vi "Simulation Configuration Read.vi"(8 "error in (no error)":errorcluster, 10 "configuration":path=path "simulation configuration.ini", 11 "simulation configuration":T1={"maxTime"=5.0, "enableVisualization"=TRUE, "statechart"=path "iRobot Navigation State Machine.vi", "environment"=path "iRobot Navigation State Machine.vi", "record"=path "Simulation Record.xml", "autograde?"=TRUE, "interactive?"=FALSE, "feedback mode"=enum."debug navigation"}) -> (0 "error out":errorcluster, 3 "simulation configuration":T1={"maxTime"=5.0, "enableVisualization"=TRUE, "statechart"=path "iRobot Navigation State Machine.vi", "environment"=path "iRobot Navigation State Machine.vi", "record"=path "Simulation Record.xml", "autograde?"=TRUE, "interactive?"=FALSE, "feedback mode"=enum."debug navigation"})   [LabVIEW 2013]
uses:
  CyberSim interface/Simulation Configuration.ctl
  autograder/feedbackMode.ctl
  <vilib>/Utility/config.llb/Read Key (Path).vi
  <vilib>/Utility/config.llb/Read Key (U32).vi
  <vilib>/Utility/config.llb/NI_LVConfig.lvlib
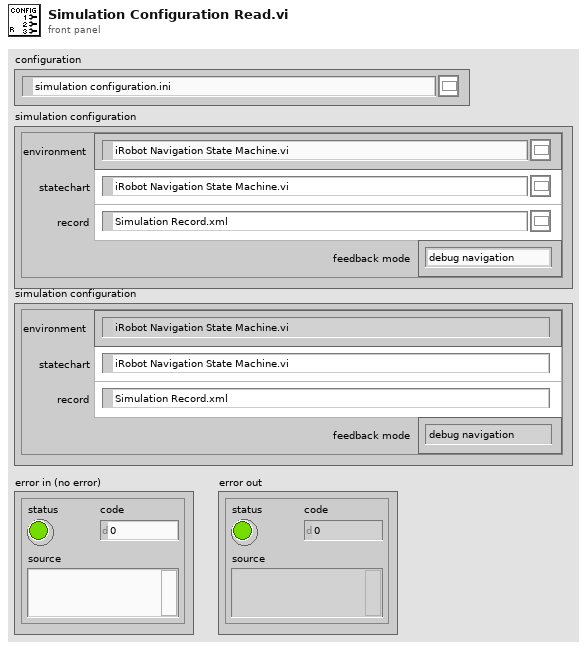
[diagram p1: front panel]
types:
  T1 = typedef "Simulation Configuration.ctl" = cluster{"maxTime":sgl, "enableVisualization":bool, "statechart":path, "environment":path, "record":path, "autograde?":bool, "interactive?":bool, "feedback mode":T2}
  T2 = typedef "feedbackMode.ctl" = enum32{"debug navigation", "debug hill climb", "autograde navigation", "autograde hill climb"}
  T3 = typedef "NI_LVConfig.lvlib/Config Data RefNum.ctl" = refnum<k1>
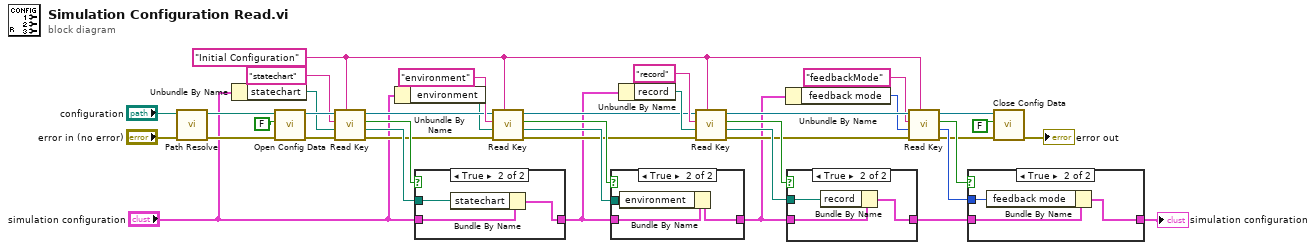
[diagram p0: block diagram]
diagram:
  w13 = "Initial Configuration" ("section")
  n1 = call "Path Resolve.vi"("Error In"="error in (no error)", "absolute or relative path"="configuration") -> ("Error Out"=w37:errorcluster, "resolved path"=w39:path)  [unwired: 8 in]
  n2 = Unbundle By Name("simulation configuration") -> ("statechart"=w21:path)
  n3 = call <vilib>:"Open Config Data.vi"("error in (no error)"=w37, "create file if necessary (T)"=FALSE, "configuration file path"=w39) -> ("error out"=w36:errorcluster, "refnum"=w35:T3)  [unwired: 6 in, 1 out]
  n4 = call-poly <vilib>:"Read Key.vi"("section"=w13, "error in (no error)"=w36, "default value"=w21, "key"="statechart" ("string key"), "refnum"=w35) -> ("error out"=w23:errorcluster, "value"=w31:path, "found?"=w32:bool, "refnum out"=w24:T3)  [unwired: 3 in]
  n5 = Unbundle By Name("simulation configuration") -> ("environment"=w20:path)
  n6 = case shown="True" w32 {
    tunnel: w31 -> [_ w43]
    tunnel: "simulation configuration" -> [w40 w42]
    tunnel: [w40 w41] -> w2
    frame False {
    }
    frame True {
      n7 = Bundle By Name(cluster=w42, "statechart"=w43) -> (w41:T1)
    }
  }
  n8 = call-poly <vilib>:"Read Key.vi"("section"=w13, "error in (no error)"=w23, "default value"=w20, "key"="environment" ("string key"), "refnum"=w24) -> ("error out"=w3:errorcluster, "value"=w29:path, "found?"=w30:bool, "refnum out"=w4:T3)  [unwired: 3 in]
  n9 = case shown="True" w30 {
    tunnel: w29 -> [_ w47]
    tunnel: w2 -> [w44 w46]
    tunnel: [w44 w45] -> w1
    frame False {
    }
    frame True {
      n10 = Bundle By Name(cluster=w46, "environment"=w47) -> (w45:T1)
    }
  }
  n11 = Unbundle By Name(w2) -> ("record"=w18:path)
  n12 = call-poly <vilib>:"Read Key.vi"("section"=w13, "error in (no error)"=w3, "default value"=w18, "key"="record", "refnum"=w4) -> ("error out"=w14:errorcluster, "value"=w16:path, "found?"=w17:bool, "refnum out"=w15:T3)  [unwired: 3 in]
  n13 = Unbundle By Name(w1) -> ("feedback mode"=w11:T2)
  n14 = case shown="True" w17 {
    tunnel: w16 -> [_ w51]
    tunnel: w1 -> [w48 w50]
    tunnel: [w48 w49] -> w9
    frame False {
    }
    frame True {
      n15 = Bundle By Name(cluster=w50, "record"=w51) -> (w49:T1)
    }
  }
  n16 = call-poly <vilib>:"Read Key.vi"("section"=w13, "error in (no error)"=w14, "default value"=w11, "key"="feedbackMode", "refnum"=w15) -> ("error out"=w5:errorcluster, "value"=w8:u32, "found?"=w10:bool, "refnum out"=w6:T3)  [unwired: 3 in]
  n17 = case shown="True" w10 {
    tunnel: w8 -> [_ w55]
    tunnel: w9 -> [w52 w54]
    tunnel: [w52 w53] -> w7
    frame False {
    }
    frame True {
      n18 = Bundle By Name(cluster=w54, "feedback mode"=w55) -> (w53:T1)
    }
  }
  "simulation configuration" <- w7
  n19 = call <vilib>:"Close Config Data.vi"("error in (no error)"=w5, "write file if changed (T)"=FALSE, "refnum"=w6) -> ("error out"=→"error out":errorcluster)  [unwired: 7 in, 1 out]
